vi "S2C_ExeScriptResetLoop.vi"(8 "Error In":errorcluster, 10 "Loops":i32, 11 "Loop?":bool) -> (0 "Error Out":errorcluster)   [LabVIEW 2015]
doc: "Resets relevant controls at the termination of execution, and displays the results banner."
uses:
  Globals/S2C_Globals.vi
  Globals/S2C_GlobalMenus.vi
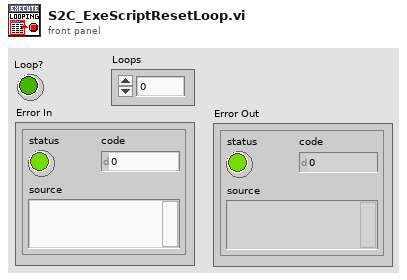
[diagram p1: front panel]
types:
  T1 = cluster{"Foreground Color":u32, "Background Color":u32}
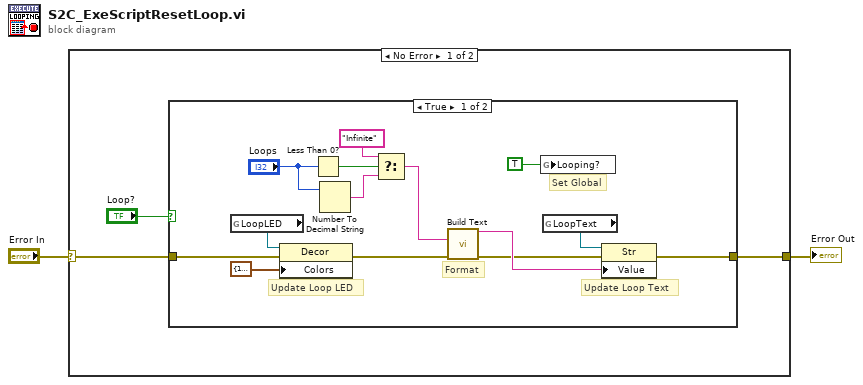
[diagram p0: block diagram]
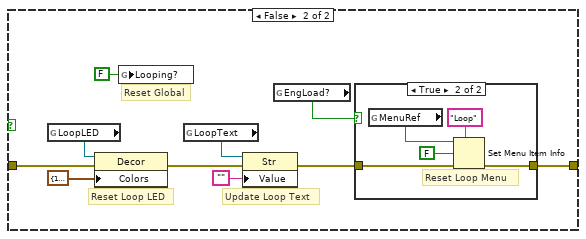
[diagram p2: hidden frame]
diagram:
  n1 = case shown="No Error" "Error In" {
    selector: "Error In" -> [w5 w36]
    tunnel: [w3 w36] -> w1
    frame No Error {
      n2 = case shown="True" "Loop?" {
        tunnel: w5 -> [w18 w26]
        tunnel: [w14 w28] -> w3
        frame True {
          # "Format"
          # "Update Loop Text"
          # "Set Global"
          # "Update Loop LED"
          n3 = global read "S2C_Globals.vi" "LoopLED"() -> (w19:refnum<vi>)
          n4 = property class="Decor"(reference=w19, error in=w18, "Colors"=T1 {"Foreground Color"=16711680, "Background Color"=16711680} ("Red")) -> (error out=w13:errorcluster)  [unwired: 1 out]
          n5 = Less Than 0?(x="Loops") -> (x < 0?=w11:bool)
          n6 = Number To Decimal String(number="Loops") -> (decimal integer string=w10:string)  [unwired: 1 in]
          n7 = Select(t="Infinite", s=w11, f=w10) -> (s? t:f=w8:string)
          n8 = call "Build Text"("Cnt"=w8, "error in (no error)"=w13) -> ("Result"=w7:string, "error out"=w6:errorcluster)  [unwired: 12 in]
          n9 = global write "S2C_Globals.vi" "Looping?"(TRUE ("Looping?")) -> ()
          n10 = global read "S2C_Globals.vi" "LoopText"() -> (w15:refnum<vi>)
          n11 = property class="Str"(reference=w15, error in=w6, "Value"=w7) -> (error out=w14:errorcluster)  [unwired: 1 out]
        }
        frame False {
          # "Update Loop Text"
          # "Reset Global"
          # "Reset Loop LED"
          n12 = global read "S2C_Globals.vi" "LoopLED"() -> (w27:refnum<vi>)
          n13 = property class="Decor"(reference=w27, error in=w26, "Colors"=T1 {"Foreground Color"=16777216, "Background Color"=16777216} ("Trans")) -> (error out=w22:errorcluster)  [unwired: 1 out]
          n14 = global write "S2C_Globals.vi" "Looping?"(FALSE ("Looping?")) -> ()
          n15 = global read "S2C_Globals.vi" "LoopText"() -> (w23:refnum<vi>)
          n16 = property class="Str"(reference=w23, error in=w22, "Value"="") -> (error out=w21:errorcluster)  [unwired: 1 out]
          n17 = global read "S2C_Globals.vi" "EngLoad?"() -> (w24:bool)
          n18 = case shown="True" w24 {
            tunnel: [w30 w32] -> w28
            tunnel: w21 -> [w30 w31]
            frame False {
              # "Running under Op Load"
            }
            frame True {
              # "Reset Loop Menu"
              n19 = global read "S2C_GlobalMenus.vi" "MenuRef"() -> (w34:refnum<k9>)
              n20 = Set Menu Item Info(6:FALSE ("checked"), 7:"Loop" ("item tag"), 8:w31, 11:w34) -> (0:w32:errorcluster)  [unwired: 3 in, 1 out]
            }
          }
        }
      }
    }
    frame Error {
    }
  }
  "Error Out" <- w1
